vi "Data File_Folder Search.vi"() -> ()   [LabVIEW 2018]
uses:
  <vilib>/KATE/Files/File Utils.lvlib
panel:
  in  "Main Tab":enum32{"Control", "Maint"}(tab)
  out "Active":bool
  in  "File_Folder Tab":enum32{"Files", "Folders"}(tab)
  out "File List":path[](array[path])
  out "Folder List":path[](array[path])
  in  "List Files in Sub Folders":bool
  in  "Search Pattern":string
  in  "Search Folder":path
  out "File Count":i32
  in  "Search":bool
  out "Folder Count":i32
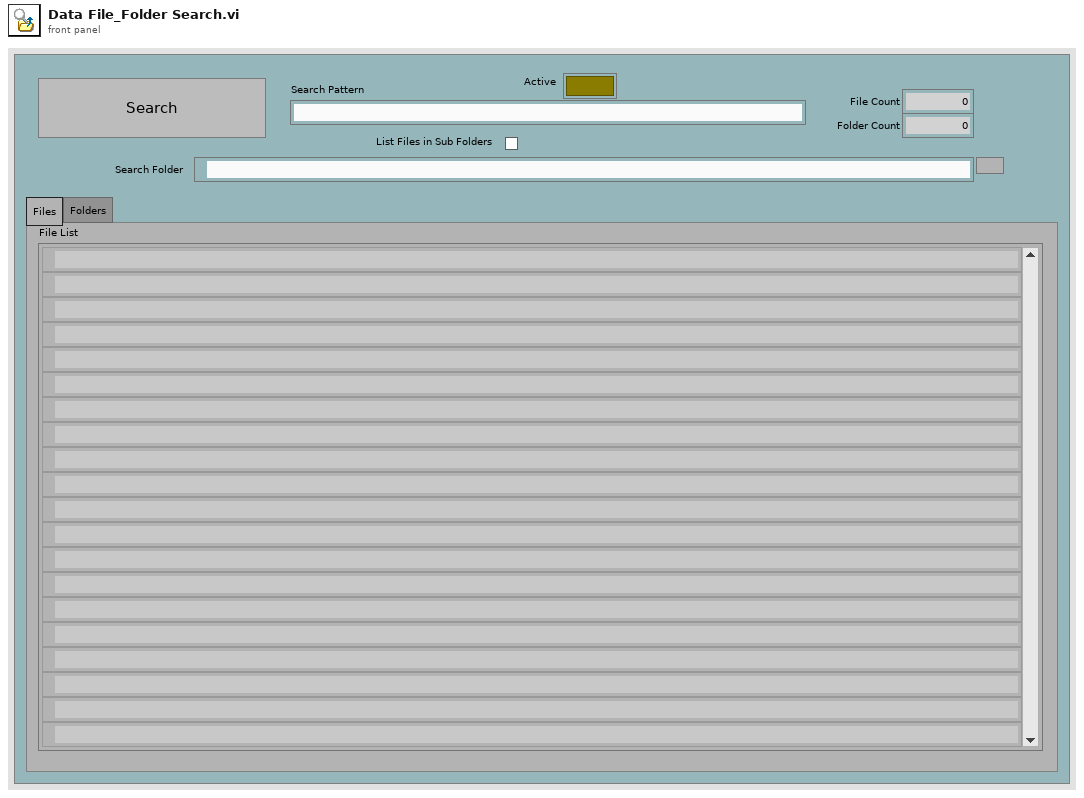
[diagram p1: front panel]
types:
  T1 = enum32{"invalid app kind", "Development System", "Run Time System", "Student Edition", "Embedded LabVIEW", "Evaluation", "Custom"}
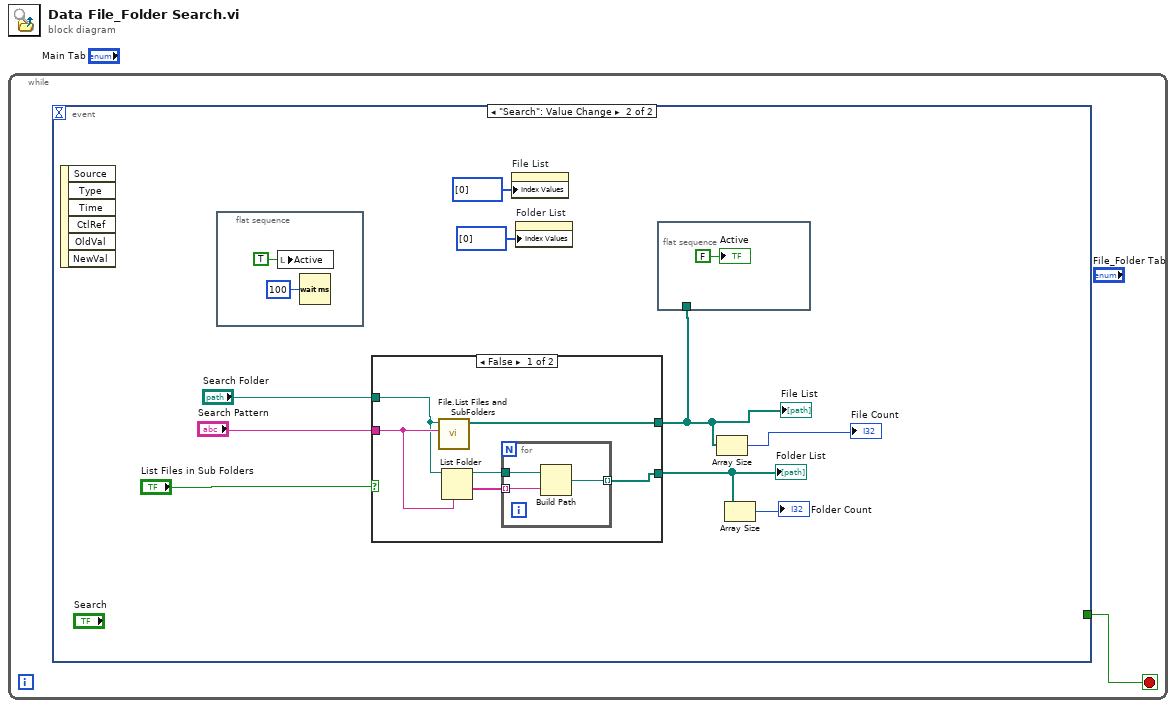
[diagram p0: block diagram]
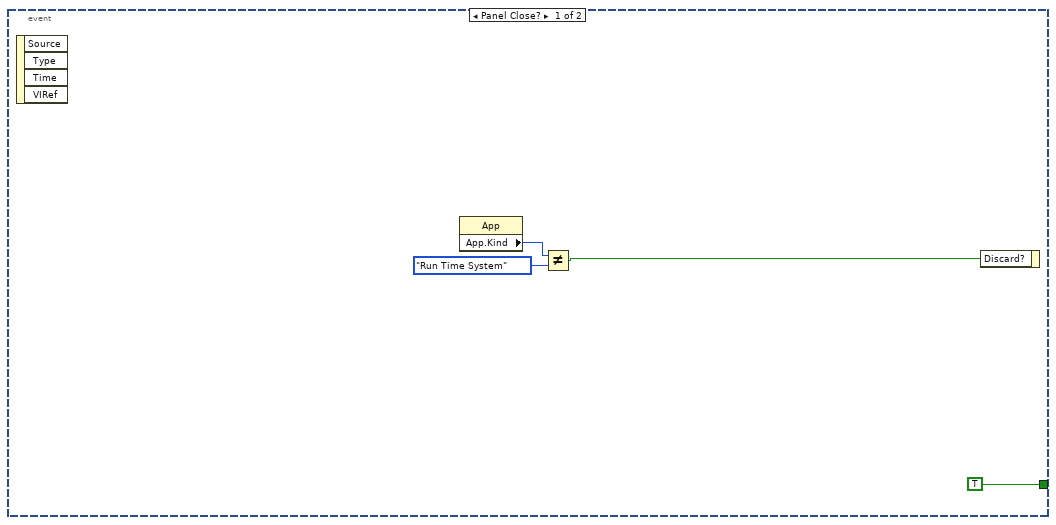
[diagram p2: hidden frame]
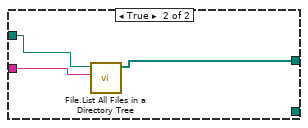
[diagram p3: hidden frame]
diagram:
  n1 = while {
    stop <- w1 stop-if-true
    n2 = event shown="[1] \"Search\": Value Change" {
      selector: _ -> [_ _]
      dyn-events: _ -> [_ _]
      timeout: _ -> [_ _]
      tunnel: [TRUE _] -> w1
      event Panel Close? {
        n3 = event-data() -> ()  [unwired: 1 in, 4 out]
        n4 = property class="App"() -> ("App.Kind"=w4:T1)  [unwired: 2 in, 2 out]
        n5 = Not Equal?(x=w4, y=T1."Run Time System") -> (x != y?=w2:bool)
        n6 = event-data("Discard?"=w2) -> ()  [unwired: 1 in, 1 out]
      }
      event "Search": Value Change {
        n7 = event-data() -> ()  [unwired: 1 in, 6 out]
        n8 = flat-sequence {
          frame #0 {
            n9 = local write "Active"(TRUE ("Active")) -> ()
            n10 = Wait (ms)(milliseconds to wait=u32 100) -> ()  [unwired: 1 out]
          }
        }
        n11 = case shown="False" "List Files in Sub Folders" {
          tunnel: [w23 w27] -> w8
          tunnel: [w18 _] -> w10
          tunnel: "Search Pattern" -> [w22 w28]
          tunnel: "Search Folder" -> [w21 w29]
          frame False {
            n12 = call <vilib>:"File.List Files and SubFolders.vi"("Pattern"=w22, "Folder"=w21) -> ("Files"=w23:path[])  [unwired: 7 in, 2 out]
            n13 = List Folder(path=w21, pattern=w22) -> (path out=w20:path, folder names=w19:string[])  [unwired: 2 in, 2 out]
            n14 = for {
              tunnel: w20 -> [w26]
              tunnel: w19 -> [w25] mode=indexing
              tunnel: [w24] -> w18 mode=indexing
              n15 = Build Path(base path=w26, name or relative path=w25) -> (appended path=w24:path)
            }
          }
          frame True {
            n16 = call <vilib>:"File.List All Files in a Directory Tree.vi"("Pattern"=w28, "Folder"=w29) -> ("Files"=w27:path[])  [unwired: 8 in, 1 out]
          }
        }
        "Folder List" <- w10
        "File List" <- w8
        n17 = property on="File List" class="Arr (strict)"("Index Values"=u32[] [0]) -> ()  [unwired: 2 in, 2 out]
        n18 = property on="Folder List" class="Arr (strict)"("Index Values"=u32[] [0]) -> ()  [unwired: 2 in, 2 out]
        n19 = flat-sequence {
          tunnel: w8 -> [_]
          frame #0 {
            "Active" <- FALSE ("Active")
          }
        }
        n20 = Array Size(array=w8) -> (size(s)=→"File Count":i32)
        n21 = Array Size(array=w10) -> (size(s)=→"Folder Count":i32)
      }
    }
  }
